vi "LV to ITX XY2 AutoPlot.vi"(6 "input command string":string="Display/R '#wave#'\nAppendToGraph '#wave#'\nLabel bottom \"#labelX#\"\nLabel left \"#labelY#\"\nModifyGraph rgb('#wave#')=(#r#,#g#,#b#)\n\\\\s('#wave#') #label#\nModifyGraph mirror(bottom)=1\nModifyGraph width=216\nModifyGraph height={Aspect,0.6}\nModifyGraph Log(bottom)=#bottomlog#\nModifyGraph Log(left)=#leftlog#", 8 "error in":errorcluster, 9 "Notes":string, 10 "Data (Dictionary)":T1[](array[typedef]), 11 "path":path=path "C:/") -> (0 "error out":errorcluster, 3 "file out":path)   [LabVIEW 2019, in "Data.ITX.lvclass"]
doc: "Write data to ITX file. This AutoPlot VI adds commands to automatically create a graph in Igor to quickly view your data.\n\n-- path: base path to save data\n-- filename: base filename\n-- Notes: add any notes here to help you remember what experiment you did\n-- Data: Cluster array\n It is recommended that you make the first cluster an array of timestamps\n-- wavenames: Give each data array a unique name such as \"time, bias, current,...\"zz\n-- X,Y Labels: For plotting in Igor. Can be ignored.\n-- X,Y Log: Do you wan to show X or Y on Log scale in Igor?"
uses:
  Data.ITX.lvclass
  Data/Data.lvclass
  Data/Typedefs/File Type--enum.ctl
  Data/Typedefs/Dictionary--cluster.ctl
panel:
  in  "X,Y Log":i32[](array[numeric])
  in  "X,Y Labels":string[](array[string])=["x label", "y label"]
  # "Below are relevant for creating graphs in Igor"
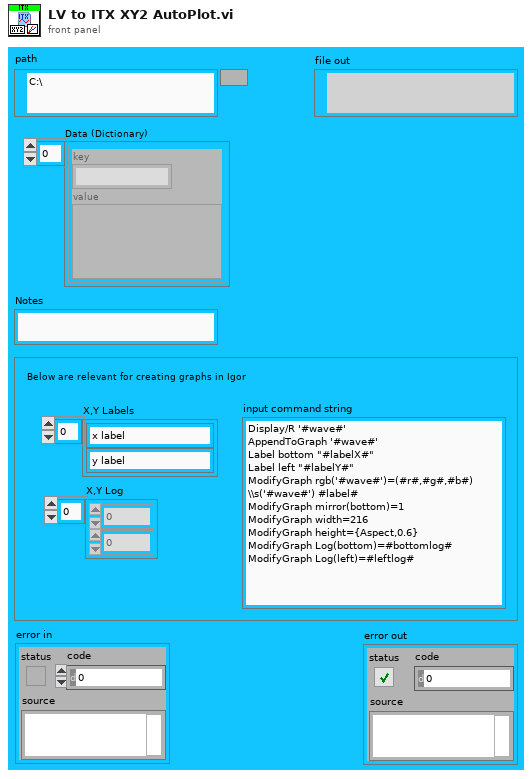
[diagram p1: front panel]
types:
  T1 = typedef "Data.lvclass/Dictionary--cluster.ctl" = cluster{"key":string, "value":variant}
  T2 = typedef "Data.lvclass/File Type--enum.ctl" = enum16{"DAT", "ITX", "HDF5", "TDMS", "VI", "PGSQL"}
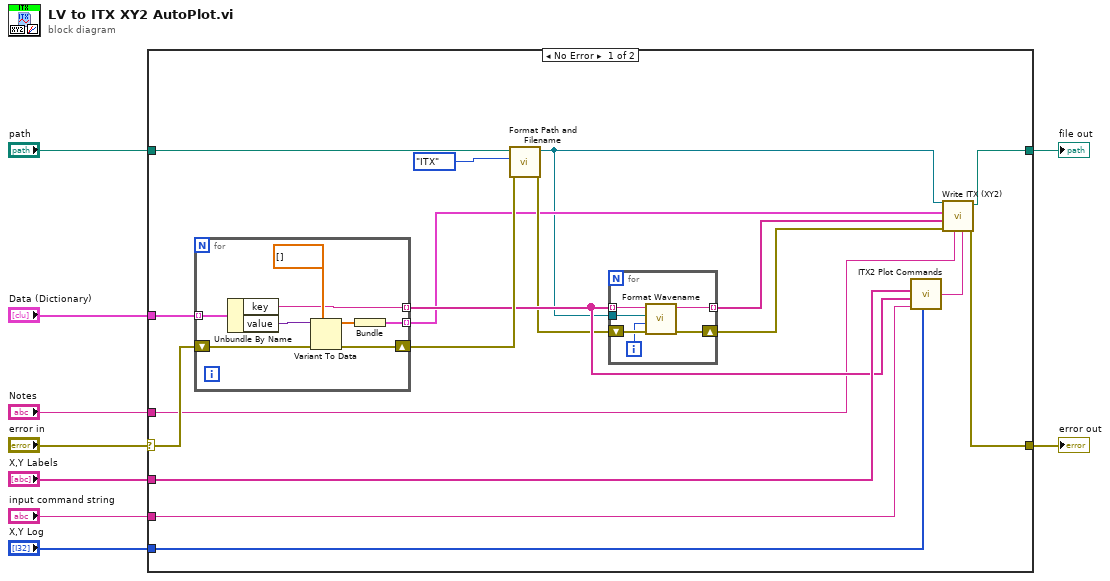
[diagram p0: block diagram]
diagram:
  n1 = case shown="No Error" "error in" {
    selector: "error in" -> [w21 w43]
    tunnel: "path" -> [w27 w42]
    tunnel: "X,Y Labels" -> [w26 _]
    tunnel: [w25 w42] -> w7
    tunnel: "X,Y Log" -> [w24 _]
    tunnel: "input command string" -> [w23 _]
    tunnel: [w13 w43] -> w4
    tunnel: "Data (Dictionary)" -> [w22 _]
    tunnel: "Notes" -> [w16 _]
    frame No Error {
      n2 = for {
        tunnel: w22 -> [w41] mode=indexing
        tunnel: [w35] -> w12 mode=indexing
        shift-right: [w36] -> w19
        shift-left: w21 -> [w39]
        tunnel: [w34] -> w18 mode=indexing
        n3 = Unbundle By Name(w41) -> ("key"=w34:string, "value"=w40:variant)
        n4 = Variant To Data(error in=w39, type=dbl[] [], Variant=w40) -> (data=w37:dbl[], error out=w36:errorcluster)
        n5 = Bundle(w37) -> (w35:cluster{dbl[]})  [unwired: 1 in]
      }
      n6 = call "Format Path and Filename.vi"("error in"=w19, 10:File_Type--enum."ITX" ("Type (TDMS)"), "Data in"=w27) -> ("error out"=w14:errorcluster, "Data out"=w10:refnum<class "Data.lvclass">)  [unwired: 7 in]
      n7 = for {
        tunnel: w18 -> [w33] mode=indexing
        shift-right: [w31] -> w15
        shift-left: w14 -> [w32]
        tunnel: [w30] -> w11 mode=indexing
        tunnel: w10 -> [w28]
        i -> [w29]
        n8 = call "Format Wavename.vi"("error in (no error)"=w32, "Index"=w29, "Path"=w28, "Name"=w33) -> ("error out"=w31:errorcluster, "Formatted wavename"=w30:string)  [unwired: 6 in]
      }
      n9 = call "ITX2 Plot Commands.vi"("X,Y Log"=w24, "input string"=w23, "Plot labels"=w18, "X,Y Labels"=w26) -> ("result string"=w17:string)  [unwired: 2 in]
      n10 = call "Write ITX (XY2).vi"("Commands"=w17, "Notes"=w16, "error in"=w15, "Wavenames"=w11, "array of clusters"=w12, "filename"=w10) -> ("error out"=w13:errorcluster, "file"=w25:path)  [unwired: 4 in]
    }
    frame Error {
    }
  }
  "file out" <- w7
  "error out" <- w4
